vi "Build Tag Path.vi"(8 "error in":errorcluster, 9 "Asset Tag":string, 10 "Asset Name":string, 11 "All Assets List":refnum<class "NI SystemLink Asset.lvclass">[](array[class])) -> (0 "error out":errorcluster, 2 "Asset Tag Path":string, 3 "All Assets List":refnum<class "NI SystemLink Asset.lvclass">[](array[class]))   [LabVIEW 2020, in "NI SystemLink Asset.lvclass"]
doc: "Constructs a tag path based on the asset you specify.\nInput: Asset Name, Tag Name, Array of asset model objects\nOutput: Asset Tag Path: Asset.<vendor_name/vendor_number><model_name/model_number><serial_number>.tag_name eg: Asset.NI_PXIe-8840_Quad-Core--SN-030DDB85--MAC-00-80-2F-25-6F-FD.Health.CPU.0.UsePercentage"
uses:
  NI SystemLink Asset.lvclass
  NI SystemLink Asset.lvclass/NI SystemLink Asset.ctl
  <vilib>/Utility/error.llb/Error Cluster From Error Code.vi
  <vilib>/ErrorRing/Error Ring.xnode
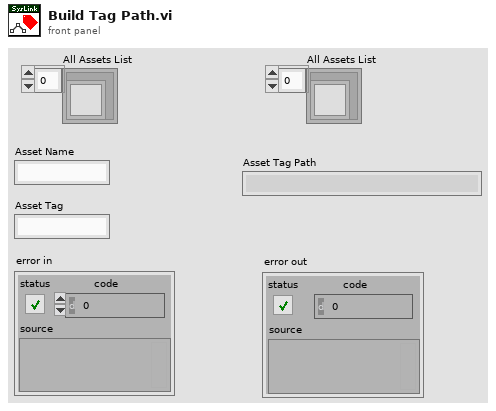
[diagram p1: front panel]
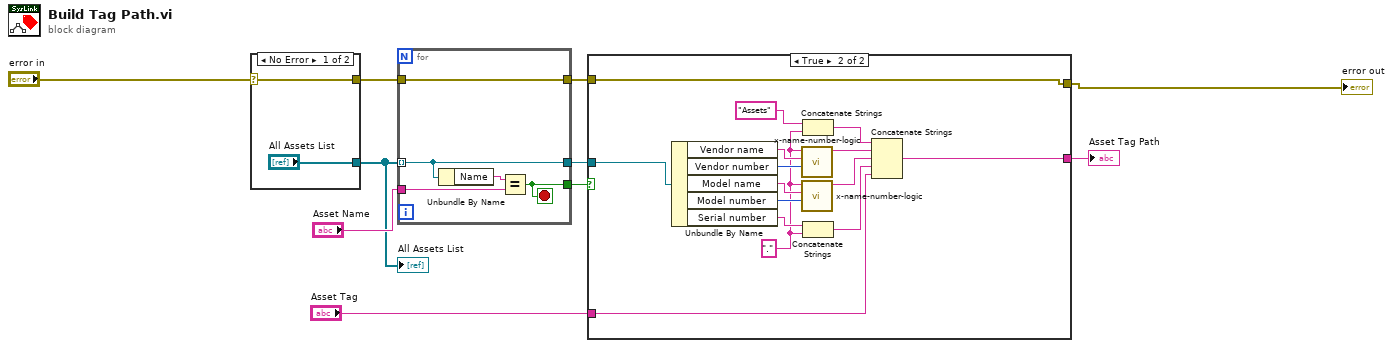
[diagram p0: block diagram]
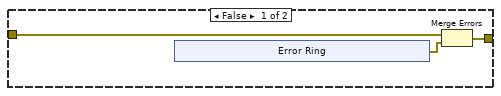
[diagram p2: hidden frame]
diagram:
  n1 = case shown="No Error" "error in" {
    selector: "error in" -> [w11 w13]
    tunnel: ["All Assets List" _] -> w7
    tunnel: [w11 w13] -> w6
    frame No Error {
    }
    frame Error {
    }
  }
  "All Assets List" <- w7
  n2 = for {
    tunnel: w7 -> [w17] mode=indexing
    tunnel: "Asset Name" -> [w15]
    tunnel: [w17] -> w5
    tunnel: w6 -> [w16]
    tunnel: [w16] -> w4
    tunnel: [w14] -> w2
    stop <- w14 stop-if-true
    n3 = Unbundle By Name(w17) -> ("Name"=w18:string)
    n4 = Equal?(x=w18, y=w15) -> (x = y?=w14:bool)
  }
  n5 = case shown="True" w2 {
    tunnel: w5 -> [_ w28]
    tunnel: w4 -> [w21 w41]
    tunnel: [w19 w41] -> w9
    tunnel: [_ w30] -> w3
    tunnel: "Asset Tag" -> [_ w29]
    frame False {
      n6 = xnode "Error Ring"() -> ("error out"=w20:errorcluster)
      n7 = Merge Errors(w21, w20) -> (w19:errorcluster)
    }
    frame True {
      w34 = "." ("string")
      n8 = Unbundle By Name(w28) -> ("Vendor name"=w37:string, "Vendor number"=w36:i64, "Model name"=w39:string, "Model number"=w38:i64, "Serial number"=w35:string)
      n9 = call "x-name-number-logic.vi"("number"=w36, "name"=w37, "string in"=w34) -> ("string out"=w33:string)  [unwired: 8 in]
      n10 = call "x-name-number-logic.vi"("number"=w38, "name"=w39, "string in"=w34) -> ("string out"=w32:string)  [unwired: 8 in]
      n11 = Concatenate Strings("Assets" ("string"), w34) -> (w27:string)
      n12 = Concatenate Strings(w35, w34) -> (w31:string)
      n13 = Concatenate Strings(w27, w33, w32, w31, w29) -> (w30:string)
    }
  }
  "error out" <- w9
  "Asset Tag Path" <- w3
